vi "PixelToMicron.vi"() -> ()   [LabVIEW 2016]
doc: "PixelToMicron.vi contains the global variable <B>PixelToMicron</B>, which can be used universally across all VIs that relate to image capture and stage motion. This value should never be written to by any VI except for designated VIs which run the PixelToMicron calibration.\nNOTE: to change the value of PixelToMicron, the default value must also be changed, so the change is not lost when LabVIEW is next restarted. To learn more about how to do this, visit this link: https://knowledge.ni.com/KnowledgeArticleDetails?id=kA00Z0000019OiiSAE"
panel:
  in  "PixelToMicron":dbl=1.5866
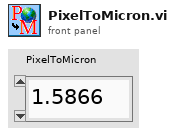
[diagram p1: front panel]
diagram:
